vi "VecBuilder_2x2Fill.vi"(8 "R1_C1":dbl, 9 "R1_C0":dbl, 10 "R0_C1":dbl, 11 "R0_C0":dbl) -> (3 "output matrix":T1)   [LabVIEW 2019, in "Trajectory_Library.lvlib"]
doc: "Creates a new LINEAR SYSTEM data cluster with the specified values. \n\n\nInputs: \n - XXX -- XXX.\n\nOutputs:\n - XXX -- XXX."
uses:
  Trajectory_Library.lvlib
  <vilib>/Analysis/Matrix/Datatypes/RealMatrix.ctl
  <vilib>/Analysis/Matrix/NI_Matrix.lvlib
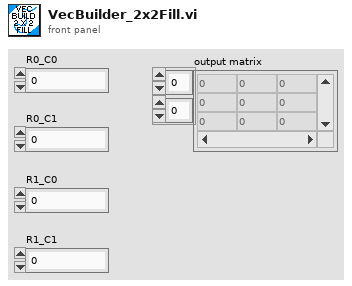
[diagram p1: front panel]
types:
  T1 = typedef "NI_Matrix.lvlib/RealMatrix.ctl" = dbl[][]
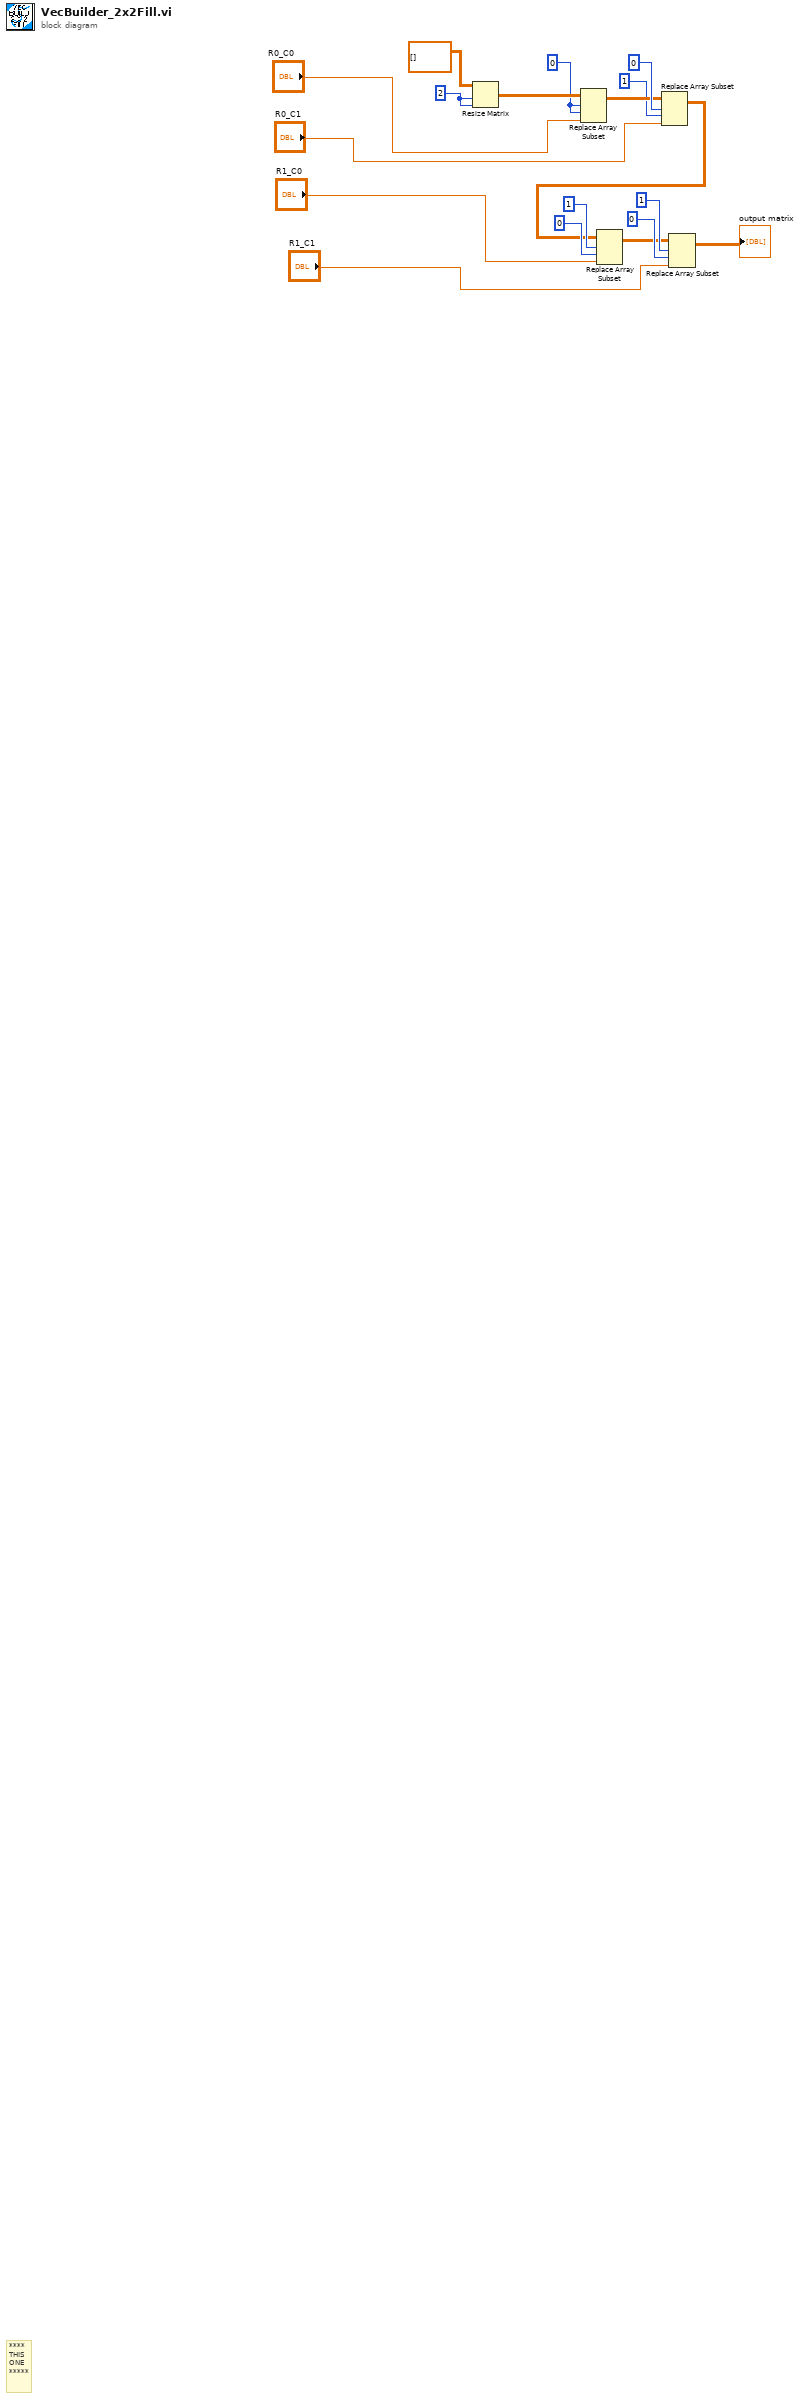
[diagram p0: block diagram]
diagram:
  w1 = 2 ("number of rows")
  w16 = 0 ("index (col)")
  # "****\nTHIS\nONE\n*****"
  n1 = Resize Matrix(1:w1, 2:w1, 4:T1 [] ("matrix")) -> (0:w17:T1)
  n2 = Replace Array Subset(array=w17, new element="R0_C0", index (row)=w16, index (col)=w16) -> (w14:T1)
  n3 = Replace Array Subset(array=w14, new element="R0_C1", index (row)=0 ("index (col)"), index (col)=1 ("disabled index (col)")) -> (w7:T1)
  n4 = Replace Array Subset(array=w7, new element="R1_C0", index (row)=1 ("index (col)"), index (col)=0 ("disabled index (col)")) -> (w8:T1)
  n5 = Replace Array Subset(array=w8, new element="R1_C1", index (row)=1 ("index (col)"), index (col)=0 ("disabled index (col)")) -> (→"output matrix":T1)
